vi "checkTempTransitionTimeElapsed.vi"(8 "error in (no error)":errorcluster, 11 "TestMonitor in":refnum<class "TestMonitor.lvclass">) -> (0 "error out":errorcluster, 1 "Wait Time Status":T1 {"Time Remaining" min=1.0 format="%.1f"}, 2 "tempTransitionTimeElapsedIsTrue":bool, 3 "TestMonitor out":refnum<class "TestMonitor.lvclass">)   [LabVIEW 2013, in "TestMonitor.lvclass"]
uses:
  TestMonitor.lvclass
  Typedefs/WaitTimeStatus.ctl
  TestMonitor.lvclass/TestMonitor.ctl
  Typedefs/AITDTTypedefs.lvlib
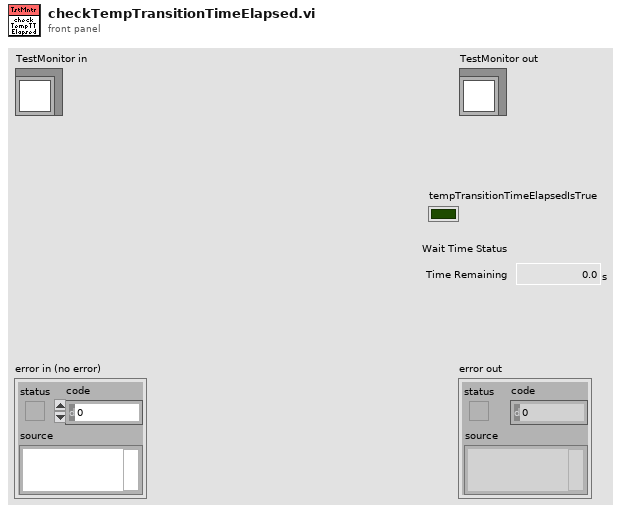
[diagram p1: front panel]
types:
  T1 = typedef "AITDTTypedefs.lvlib/WaitTimeStatus.ctl" = cluster{"Time Remaining":dbl[unit]}
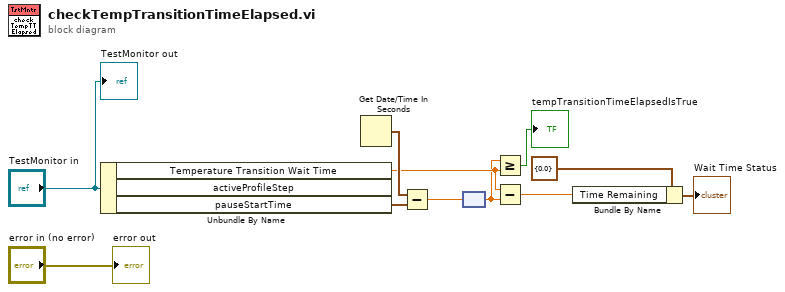
[diagram p0: block diagram]
diagram:
  n1 = Unbundle By Name("TestMonitor in") -> ("Temperature Transition Wait Time"=w3:dbl[unit], "pauseStartTime"=w8:timestamp)  [unwired: 1 out]
  n2 = Get Date/Time In Seconds() -> (seconds since 1Jan1904=w9:timestamp)
  n3 = Subtract(x=w9, y=w8) -> (x-y=w7:dbl)
  n4 = node(w7) -> (w2:dbl[unit])
  n5 = Greater Or Equal?(x=w2, y=w3) -> (x >= y?=→"tempTransitionTimeElapsedIsTrue":bool)
  n6 = Subtract(x=w3, y=w2) -> (x-y=w1:dbl[unit])
  n7 = Bundle By Name(cluster=T1 {"Time Remaining"=0.0} ("Wait Time Status"), "Time Remaining"=w1) -> (→"Wait Time Status":T1)
  "error out" <- "error in (no error)"
  "TestMonitor out" <- "TestMonitor in"
